vi "GIFAnimatedControls.vi"() -> ()   [LabVIEW 2012]
doc: "In LabVIEW 6.1, you can place animated GIF images on front panels. You also can customize a control by replacing some parts of controls with animated images. This example VI shows three visually interesting controls. No programmatic support for controlling the GIF animation exists, so you cannot synchronize or change GIFs based on the value of the control. However, several controls in the example display different custom controls for different values, such as how the VI changes between <B>TOO HIGH</B> and <B>JUST RIGHT</B>."
panel:
  out "threshold":bool=TRUE
  in  "stop":bool
  out "Hypnotic Control":dbl(knob)=6.0 scale=0.0..20.0
  in  "Disco Slide 2":dbl(slide)=4.0 scale=0.0..10.0
  in  "Disco Slide":dbl(slide)=2.0 scale=0.0..10.0
  # "Run the VI."
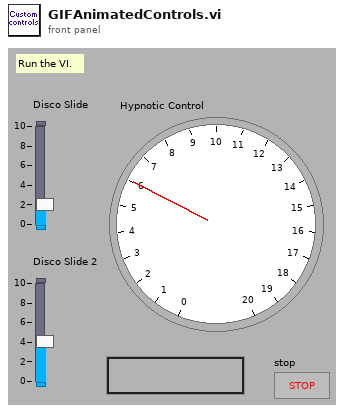
[diagram p1: front panel]
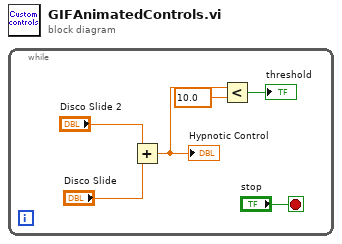
[diagram p0: block diagram]
diagram:
  n1 = while {
    stop <- "stop" stop-if-true
    n2 = Add(x="Disco Slide 2", y="Disco Slide") -> (x+y=w1:dbl)
    "Hypnotic Control" <- w1
    n3 = Less?(x=w1, y=10.0) -> (x < y?=→"threshold":bool)
  }
